vi "Array to List.vi"(10 "Array":string[](array[string])) -> (2 "List":string)   [LabVIEW 2015, in "slscsl.lvclass"]
uses:
  slscsl.lvclass
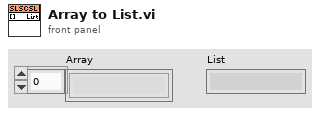
[diagram p1: front panel]
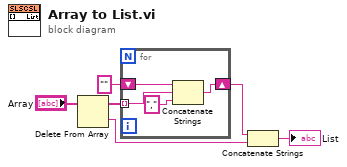
[diagram p0: block diagram]
diagram:
  n1 = Delete From Array(array="Array") -> (deleted portion=w3:string, array with subset deleted=w5:string[])  [unwired: 2 in]
  n2 = for {
    tunnel: w5 -> [w10] mode=indexing
    shift-right: [w8] -> w4
    shift-left: "" -> [w7]
    n3 = Concatenate Strings(w7, w10, "," ("element")) -> (w8:string)
  }
  n4 = Concatenate Strings(w4, w3) -> (→"List":string)
